vi "Start Acquisition.vi"(8 "error in (no error)":errorcluster, 11 "Dell Webcam in":refnum<class "Webcam.lvclass">) -> (0 "error out":errorcluster, 3 "Dell Webcam out":refnum<class "Webcam.lvclass">)   [LabVIEW 2019, in "Webcam.lvclass"]
uses:
  Webcam.lvclass
  Webcam.lvclass/Webcam.ctl
  <vilib>/vision/driver/NI_Vision_Acquisition_Software.lvlib
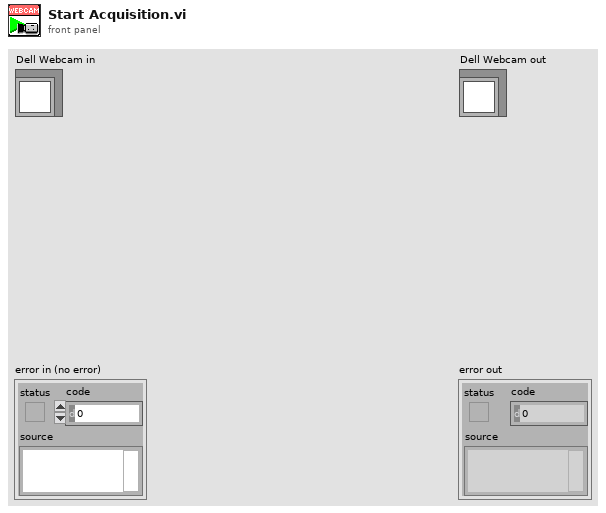
[diagram p1: front panel]
types:
  T1 = typedef "IMAQdx.ctl" = refnum<k21>
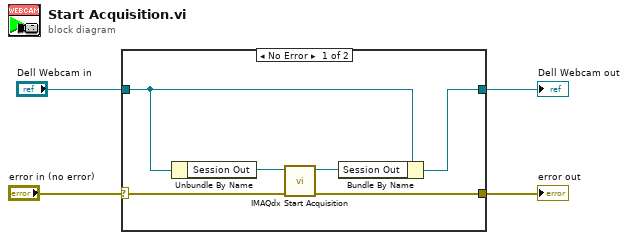
[diagram p0: block diagram]
diagram:
  n1 = case shown="No Error" "error in (no error)" {
    selector: "error in (no error)" -> [w10 w12]
    tunnel: [w9 w12] -> w3
    tunnel: [w5 w11] -> w2
    tunnel: "Dell Webcam in" -> [w7 w11]
    frame No Error {
      n2 = Unbundle By Name(w7) -> ("Session Out"=w8:T1)
      n3 = call <vilib>:"IMAQdx Start Acquisition.vi"("error in"=w10, "Session In"=w8) -> ("error out"=w9:errorcluster, "Session Out"=w6:T1)  [unwired: 8 out]
      n4 = Bundle By Name(cluster=w7, "Session Out"=w6) -> (w5:refnum<class "Webcam.lvclass">)
    }
    frame Error {
    }
  }
  "error out" <- w3
  "Dell Webcam out" <- w2
